vi "Match Messages.vi"(8 "error in (no error)":errorcluster, 11 "RemoteControl.ZMQ in":refnum<class "RemoteControl.ZMQ.lvclass">) -> (0 "error out":errorcluster, 2 "Match":bool, 3 "RemoteControl.ZMQ out":refnum<class "RemoteControl.ZMQ.lvclass">)   [LabVIEW 2019, in "RemoteControl.ZMQ.lvclass"]
uses:
  RemoteControl.ZMQ.lvclass
  \\Mac\Home/Documents/GitHub/Instrument-Framework/lvsrc/SMOs/RemoteControl/RemoteControl.lvclass
  RemoteControl/RemoteControl.lvclass/RemoteControl.ctl
  RemoteControl/RemoteControl.lvclass
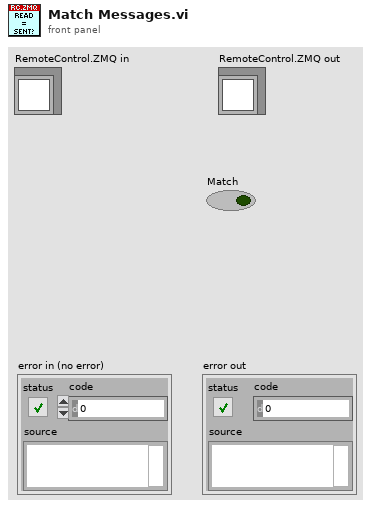
[diagram p1: front panel]
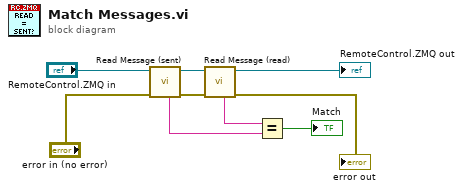
[diagram p0: block diagram]
diagram:
  n1 = call "Read Message (sent).vi"("error in (no error)"="error in (no error)", "RemoteControl in"="RemoteControl.ZMQ in") -> ("error out"=w8:errorcluster, "RemoteControl out"=w9:refnum<class "RemoteControl.ZMQ.lvclass">, "ID (Sent)"=w2:string)  [unwired: 5 in, 2 out]
  n2 = call "Read Message (read).vi"("error in (no error)"=w8, "RemoteControl in"=w9) -> ("error out"=→"error out":errorcluster, "RemoteControl out"=→"RemoteControl.ZMQ out":refnum<class "RemoteControl.ZMQ.lvclass">, "ID (Read)"=w3:string)  [unwired: 5 in, 2 out]
  n3 = Equal?(x=w3, y=w2) -> (x = y?=→"Match":bool)
